vi "Open_single_Image.vi"(6 "Image Name":string="image_input", 8 "error in (no error)":errorcluster, 10 "appended path":path, 11 "Refnum in":T1) -> (0 "error out":errorcluster, 3 "Refnum out":T1)   [LabVIEW 2021, in "Framework_lib.lvlib"]
uses:
  QMH/Framework_lib.lvlib
  <vilib>/vision/Image Controls.llb/IMAQ Image.ctl
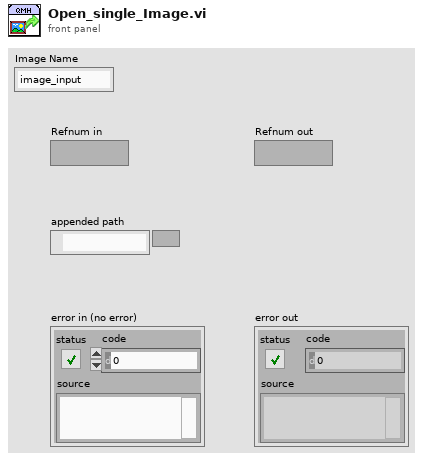
[diagram p1: front panel]
types:
  T1 = typedef "IMAQ Image.ctl" = refnum<image>
  T2 = typedef "Image Type" = u32
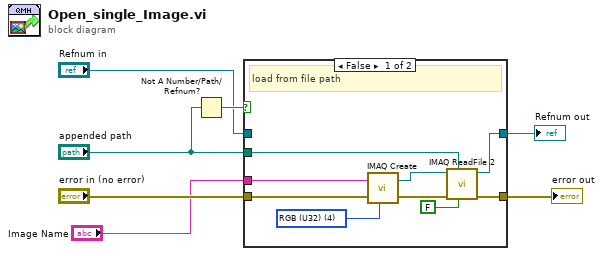
[diagram p0: block diagram]
diagram:
  n1 = Not A Number/Path/Refnum?(number/path/refnum="appended path") -> (NaN/Path/Refnum?=w4:bool)
  n2 = case shown="False" w4 {
    tunnel: [w16 w18] -> w7
    tunnel: [w14 w17] -> w6
    tunnel: "appended path" -> [w13 _]
    tunnel: "Refnum in" -> [_ w18]
    tunnel: "error in (no error)" -> [w12 w17]
    tunnel: "Image Name" -> [w8 _]
    frame False {
      w10 = T2 4 items=["Grayscale (U8)", "Grayscale (I16)", "Grayscale (SGL)", "Complex (CSG)", "RGB (U32)", "HSL (U32)", "RGB (U64)", "Grayscale (U16)"] ("Image Type")
      # "load from file path"
      n3 = call "IMAQ Create"("Image Name"=w8, "Image Type"=w10, "error in (no error)"=w12) -> ("New Image"=w11:T1, "error out"=w9:errorcluster)  [unwired: 2 in]
      n4 = call "IMAQ ReadFile 2"("Use File Path Image Type"=FALSE, "File Path"=w13, "error in (no error)"=w9, "Image"=w11) -> ("error out"=w14:errorcluster, "Image Out"=w16:T1)  [unwired: 3 in, 3 out]
    }
    frame True {
      # "reuse Imaq ref"
    }
  }
  "Refnum out" <- w7
  "error out" <- w6
